vi "Thermistor-Conversion.vi"(6 "C":dbl, 9 "B":dbl, 10 "A":dbl, 11 "Input voltage":dbl) -> (1 "Temperature (K)":dbl)   [LabVIEW 2020]
panel:
  in  "Resistor":i32=10000
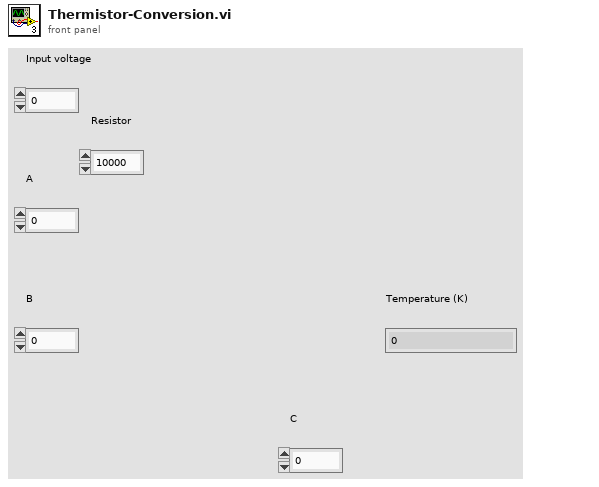
[diagram p1: front panel]
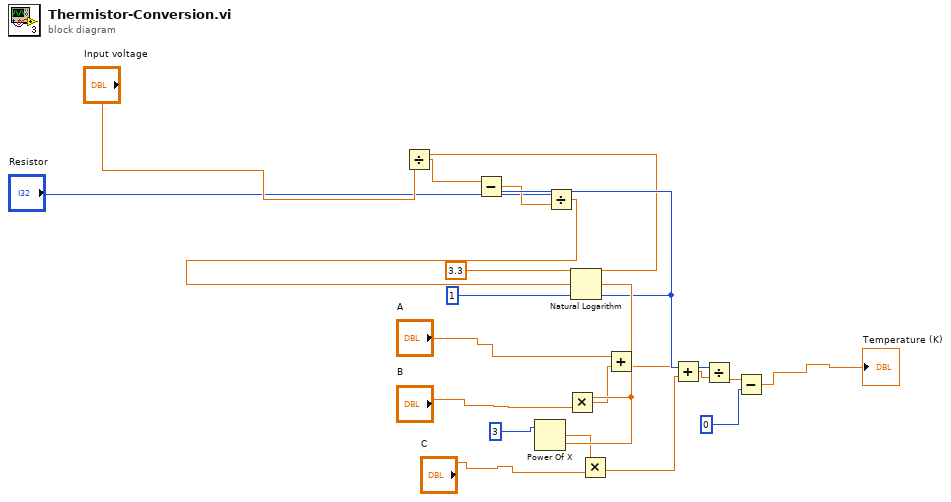
[diagram p0: block diagram]
diagram:
  w11 = 1
  n1 = Divide(x=3.3, y="Input voltage") -> (x/y=w3:dbl)
  n2 = Subtract(x=w3, y=w11) -> (x-y=w4:dbl)
  n3 = Divide(x="Resistor", y=w4) -> (x/y=w20:dbl)
  n4 = Natural Logarithm(1:w20) -> (0:w14:dbl)
  n5 = Power Of X(1:w14, 2:3) -> (0:w5:dbl)
  n6 = Multiply(x=w14, y="B") -> (x*y=w8:dbl)
  n7 = Multiply(x=w5, y="C") -> (x*y=w9:dbl)
  n8 = Add(x="A", y=w8) -> (x+y=w7:dbl)
  n9 = Add(x=w7, y=w9) -> (x+y=w10:dbl)
  n10 = Divide(x=w11, y=w10) -> (x/y=w12:dbl)
  n11 = Subtract(x=w12, y=0) -> (x-y=→"Temperature (K)":dbl)
